vi "GetBlock.vi"(9 "Line":string="2", 10 "Program Number":string="555885", 11 "Folder Name":path=path "C:/Users/me1ssv/Music/MTConnect") -> (2 "Tool Data":string="\n", 3 "Block":string)   [LabVIEW 2014]
panel:
  out "text":string
  out "appended path":path
  in  "error in":errorcluster
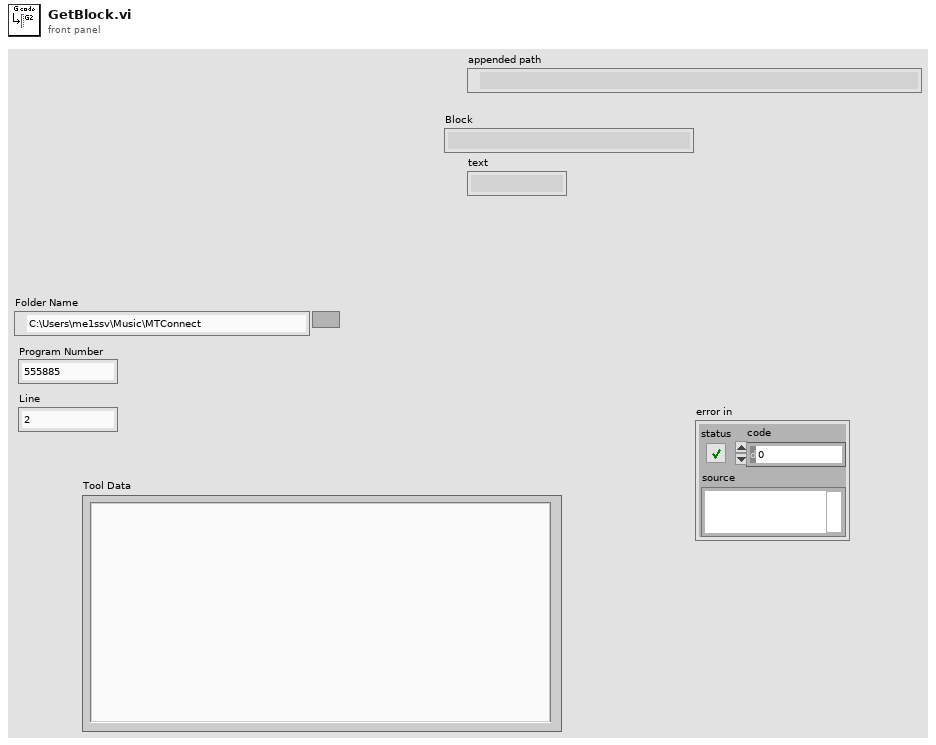
[diagram p1: front panel]
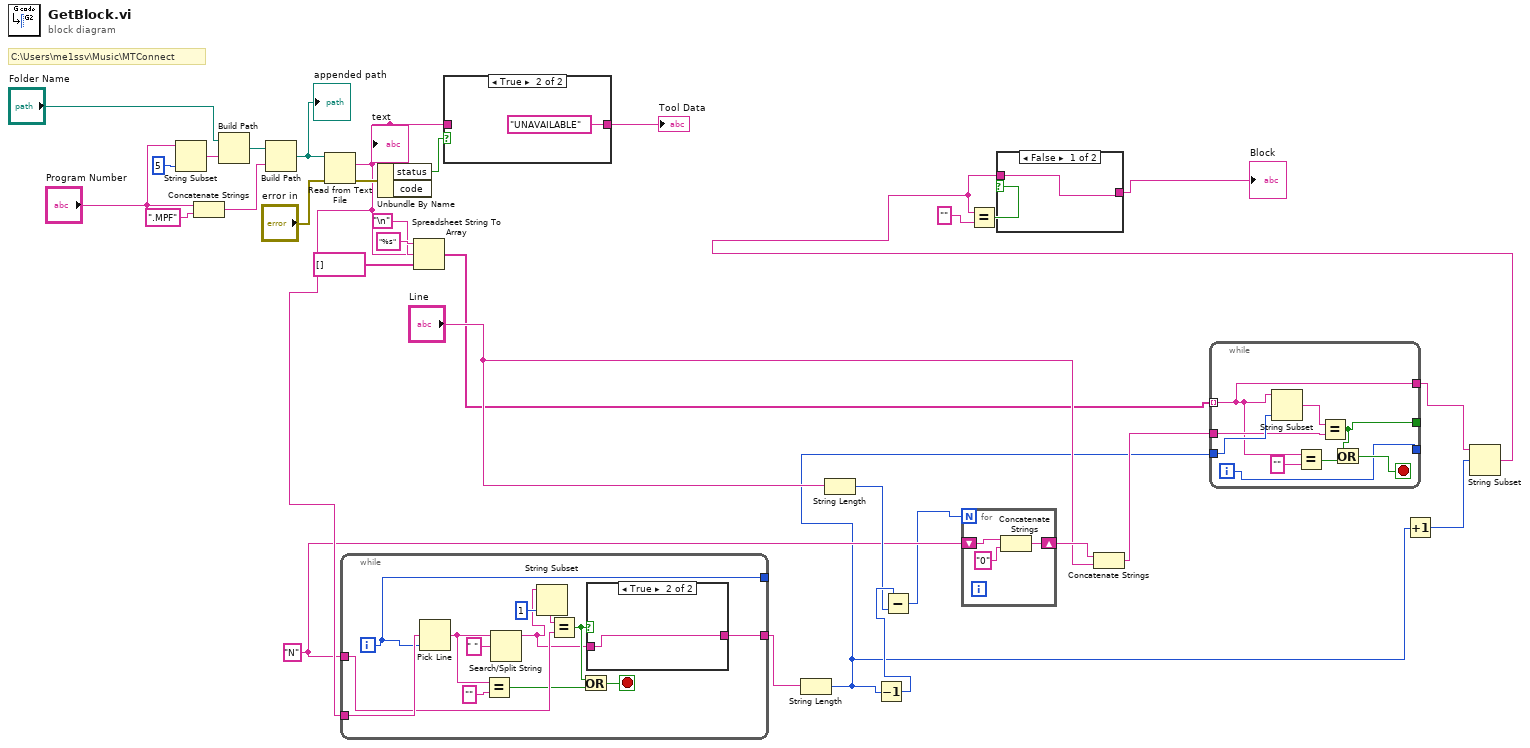
[diagram p0: block diagram]
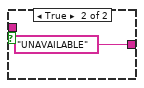
[diagram p2: hidden frame]
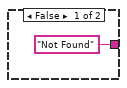
[diagram p3: hidden frame]
diagram:
  w13 = "N" ("ProgramName")
  # "C:\\Users\\me1ssv\\Music\\MTConnect"
  n1 = String Subset(string="Program Number", length (rest)=5 ("length (rest)")) -> (substring=w20:string)  [unwired: 1 in]
  n2 = Concatenate Strings("Program Number", ".MPF" ("string")) -> (w28:string)
  n3 = Build Path(base path="Folder Name", name or relative path=w20) -> (appended path=w21:path)
  n4 = Build Path(base path=w21, name or relative path=w28) -> (appended path=w32:path)
  "appended path" <- w32
  n5 = Read from Text File(file (use dialog)=w32, error in="error in") -> (text=w17:string, error out=w31:errorcluster)  [unwired: 2 in, 2 out]
  "text" <- w17
  n6 = while {
    tunnel: w17 -> [w45]
    tunnel: [w35] -> _
    tunnel: w13 -> [w42]
    tunnel: [w41] -> w16
    i -> [w35]
    stop <- w38 stop-if-true
    n7 = Pick Line(multi-line string=w45, line index=w35) -> (output string=w43:string)  [unwired: 1 in]
    n8 = Equal?(x=w43, y="") -> (x = y?=w39:bool)
    n9 = Search/Split String(string=w43, search string/char (-)=" ") -> (substring before match=w34:string)  [unwired: 1 in, 2 out]
    n10 = String Subset(string=w34, length (rest)=1 ("length (rest)")) -> (substring=w36:string)  [unwired: 1 in]
    n11 = Equal?(x=w36, y=w42) -> (x = y?=w40:bool)
    n12 = Or(x=w40, y=w39) -> (x .or. y?=w38:bool)
    n13 = case shown="True" w40 {
      tunnel: w34 -> [_ w47]
      tunnel: ["Not Found" ("output string") w47] -> w41
      frame False {
      }
      frame True {
      }
    }
  }
  n14 = Unbundle By Name(w31) -> ("status"=w23:bool)  [unwired: 1 out]
  n15 = Spreadsheet String To Array(delimiter (Tab)="\n", format string="%s", spreadsheet string=w17, array type (2D Dbl)=string[] []) -> (array=w9:string[])
  n16 = case shown="True" w23 {
    tunnel: w17 -> [w48 _]
    tunnel: [w48 "UNAVAILABLE"] -> w29
    frame False {
    }
    frame True {
    }
  }
  "Tool Data" <- w29
  n17 = String Length(string=w16) -> (length=w5:i32)
  n18 = String Length(string="Line") -> (length=w14:i32)
  n19 = Decrement(x=w5) -> (x-1=w15:i32)
  n20 = Subtract(x=w15, y=w14) -> (x-y=w12:i32)
  n21 = for {
    N: w12 -> [_]
    shift-right: [w51] -> w11
    shift-left: w13 -> [w50]
    n22 = Concatenate Strings(w50, "0" ("string")) -> (w51:string)
  }
  n23 = Concatenate Strings(w11, "Line") -> (w8:string)
  n24 = while {
    tunnel: w9 -> [w53] mode=indexing
    tunnel: w5 -> [w61]
    tunnel: w8 -> [w58]
    tunnel: [w57] -> _
    tunnel: [w54] -> _
    tunnel: [w53] -> w7
    i -> [w54]
    stop <- w55 stop-if-true
    n25 = String Subset(string=w53, length (rest)=w61) -> (substring=w59:string)  [unwired: 1 in]
    n26 = Equal?(x=w53, y="") -> (x = y?=w56:bool)
    n27 = Equal?(x=w59, y=w58) -> (x = y?=w57:bool)
    n28 = Or(x=w57, y=w56) -> (x .or. y?=w55:bool)
  }
  n29 = Increment(x=w5) -> (x+1=w6:i32)
  n30 = String Subset(string=w7, offset (0)=w6) -> (substring=w1:string)  [unwired: 1 in]
  n31 = Equal?(x=w1, y="" ("substring")) -> (x = y?=w3:bool)
  n32 = case shown="False" w3 {
    tunnel: [w62 "UNAVAILABLE"] -> w2
    tunnel: w1 -> [w62 _]
    frame False {
    }
    frame True {
    }
  }
  "Block" <- w2
